vi "MacrotoXML.vi"(1 "MacroSaveCluster":T1 {"Instructions"."Steps" min=1 max=100000 step=1; "Instructions"."Duration" min=0.001 step=0.001 format="%_6p"}, 2 "XML File Path":path) -> ()   [LabVIEW 2018]
uses:
  MacroSaveCluster.ctl
  Instructions.ctl
  Executor Files/RT/Instruction.ctl
  <vilib>/Utility/xml.llb/Write to XML File(string).vi
panel:
  # "0        2       4       6        8      10     12     14     16     18      20    22     24     26     28     30     32     34     36"
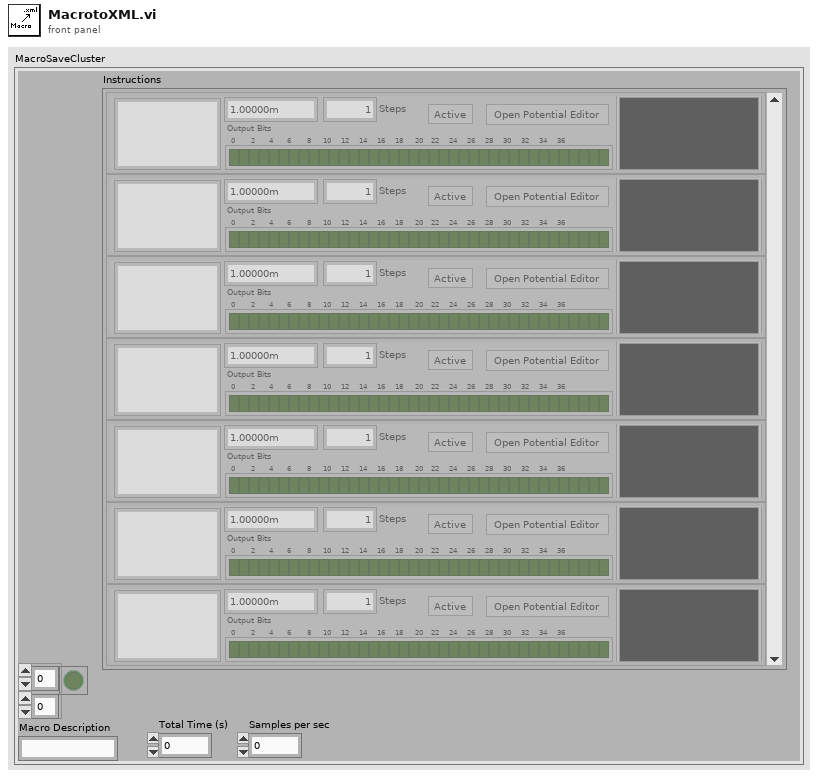
[diagram p1: front panel]
types:
  T1 = typedef "MacroSaveCluster.ctl" = cluster{"Instructions":T2, "Changes":bool[][], "Macro Description":string, "Total Time (s)":dbl, "Samples per sec":dbl}
  T2 = typedef "Instructions.ctl" = T3[]
  T3 = typedef "Instruction.ctl" = cluster{"Duration":dbl, "Comment":string, "Steps":i32, "Edit Potential":bool, "Output Bits":bool[], "Macro Path":path, "Potentials":dbl[], "Inherit?":bool}
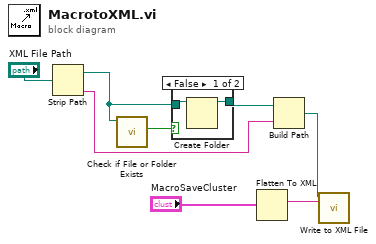
[diagram p0: block diagram]
diagram:
  n1 = Strip Path(path="XML File Path") -> (stripped path=w5:path, name=w3:string)
  n2 = call <vilib>:"Check if File or Folder Exists.vi"("path"=w5) -> ("file or folder exists?"=w7:bool)  [unwired: 8 in, 2 out]
  n3 = case shown="False" w7 {
    tunnel: w5 -> [w10 w11]
    tunnel: [w9 w11] -> w4
    frame False {
      n4 = Create Folder(path (use dialog)=w10) -> (created path=w9:path)  [unwired: 2 in, 2 out]
    }
    frame True {
    }
  }
  n5 = Flatten To XML(anything="MacroSaveCluster") -> (xml string=w8:string)
  n6 = Build Path(base path=w4, name or relative path=w3) -> (appended path=w2:path)
  n7 = call-poly <vilib>:"Write to XML File.vi"("XML Input"=w8, "XML File Path"=w2) -> ()  [unwired: 7 in, 3 out]
